vi "feed_forward.vi"(0 "Desired tension velocities [N/s]":dbl[](array[numeric]), 4 "frictionCompensationTensions":dbl[](array[numeric])=[30.0, 30.0, 30.0, 30.0, 30.0, 30.0, 30.0, 30.0, 30.0, 30.0, 30.0, 30.0, 30.0, 30.0], 5 "Use pull-only friction compensation in feedforward":bool, 6 "Motor velocities (rpm)":dbl[](array[numeric]), 7 "DesiredTensionsInAscendingMotorOrder":dbl[](array[numeric]), 8 "Use linear tension/current modle in feedforward":bool, 9 "Num Total Active Motors":i32, 10 "lastCommandedMotorCurrent":dbl[](array[numeric]), 11 "Constants LL":T1) -> (3 "feedforwardPredictedMotorCurrents":dbl[](array[numeric]))   [LabVIEW 2024]
uses:
  typeDef/constants_LL.ctl
panel:
  in  "motor velocity friction comp exponent denominator (rpm)":dbl=50.0
  # "FRICTION COMPENSATION \nVALUES BELOW. \nNOTE: Friction Comp tensions \nare passed in from outside."
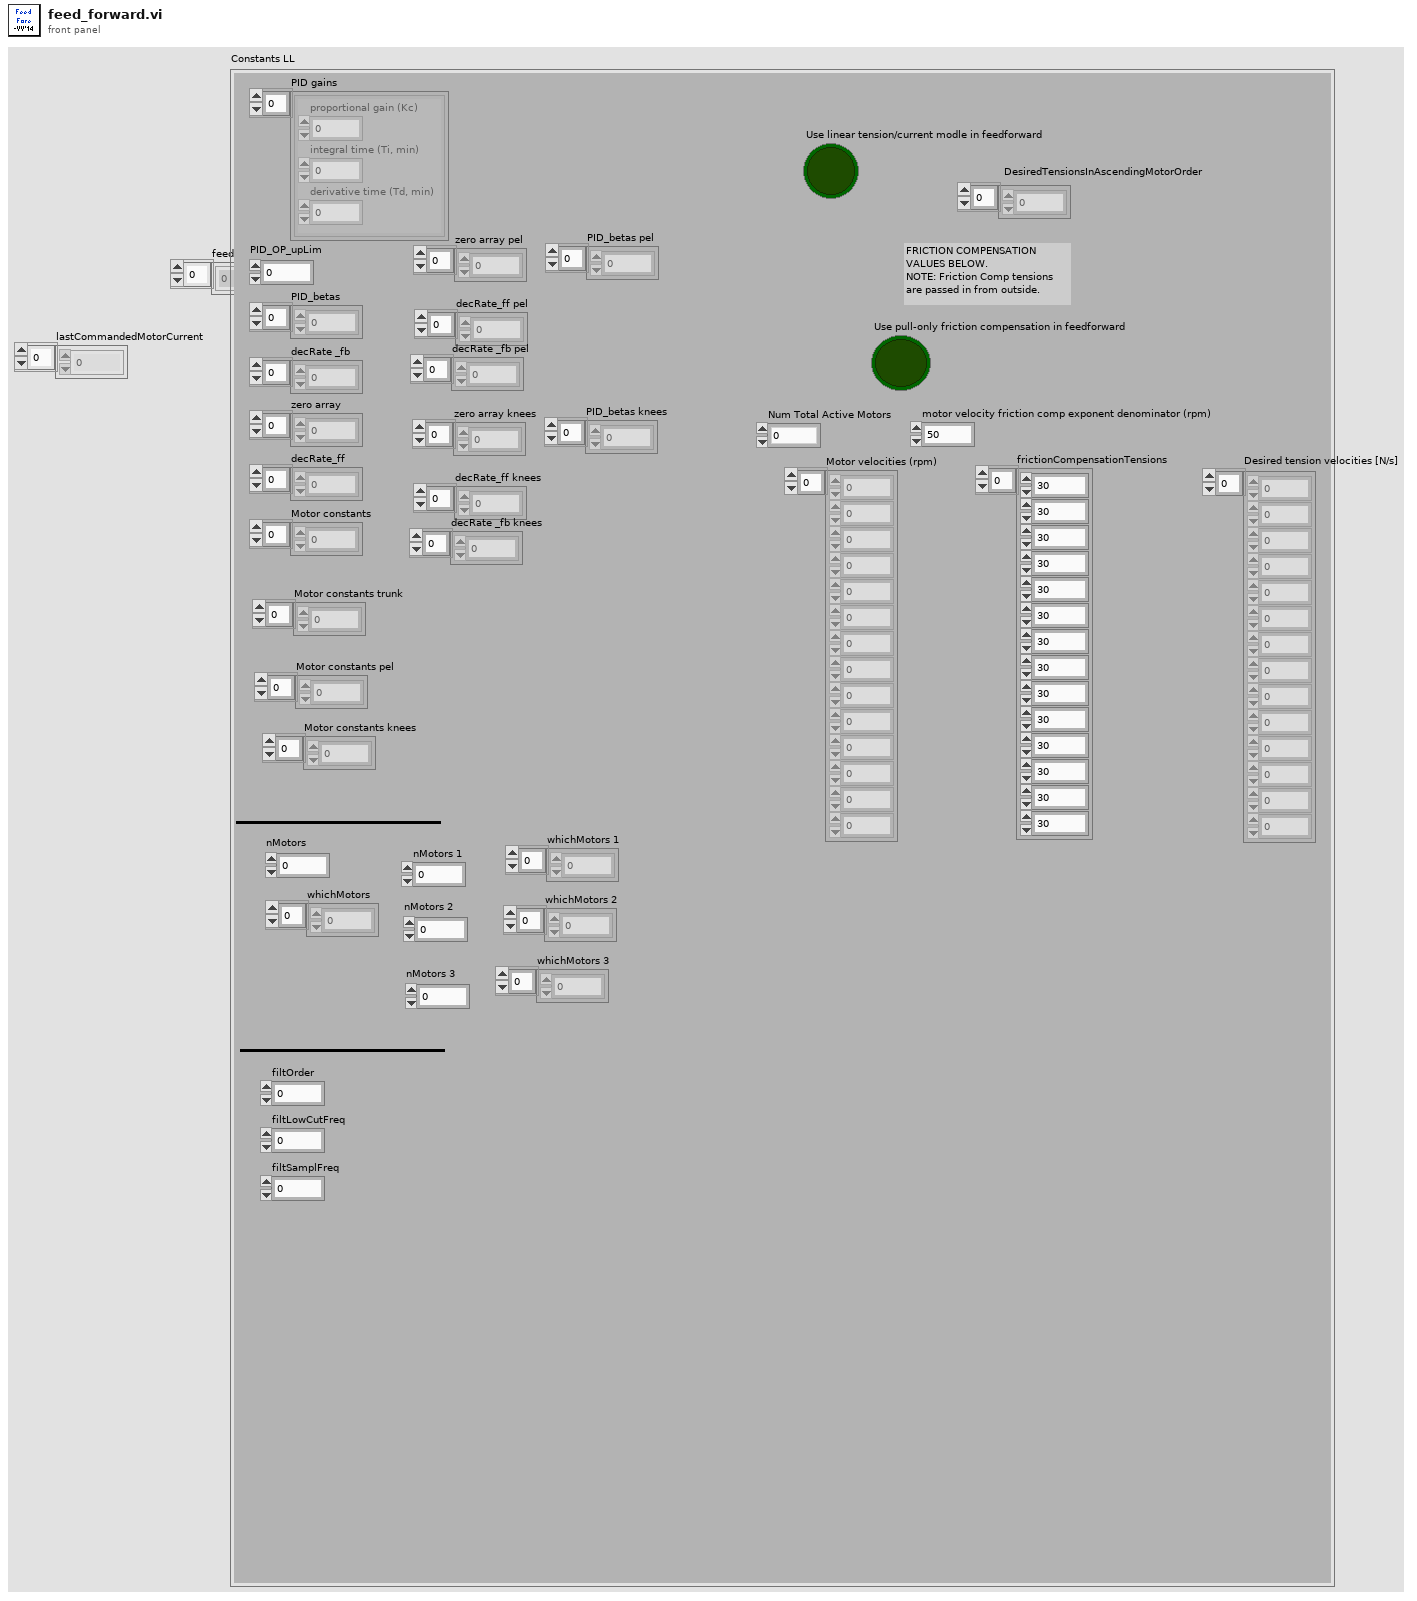
[diagram p1: front panel]
types:
  T1 = typedef "constants_LL.ctl" = cluster{"zero array":dbl[], "decRate_ff":dbl[], "Motor constants":dbl[], "PID gains":cluster{"proportional gain (Kc)":dbl, "integral time (Ti, min)":dbl, "derivative time (Td, min)":dbl}[], "decRate _fb":dbl[], "PID_OP_upLim":dbl, "nMotors":i32, "PID_betas":dbl[], "filtOrder":i32, "filtLowCutFreq":dbl, "filtSamplFreq":dbl, "whichMotors":i32[], "nMotors 1":i32, "nMotors 2":i32, "Motor constants pel":dbl[], "Motor constants trunk":dbl[], "whichMotors 1":i32[], "whichMotors 2":i32[], "zero array pel":dbl[], "decRate_ff pel":dbl[], "decRate _fb pel":dbl[], "PID_betas pel":dbl[], "whichMotors 3":i32[], "nMotors 3":i32, "Motor constants knees":dbl[], "zero array knees":dbl[], "decRate_ff knees":dbl[], "decRate _fb knees":dbl[], "PID_betas knees":dbl[]}
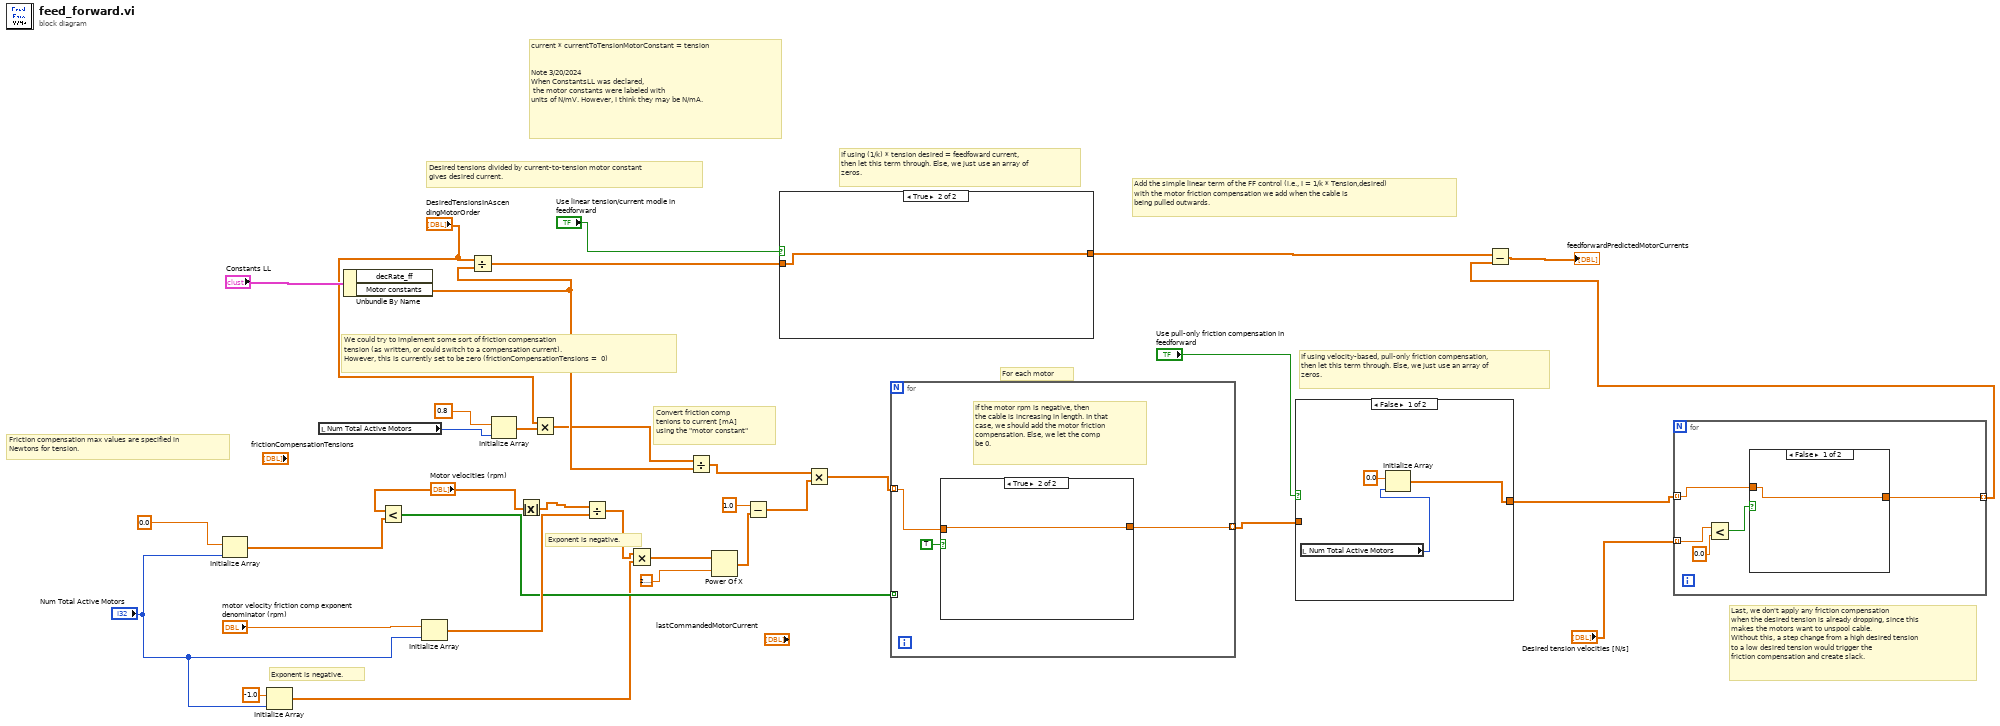
[diagram p0: block diagram]
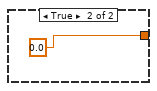
[diagram p2: hidden frame]
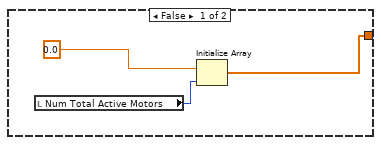
[diagram p4: hidden frame]
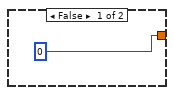
[diagram p5: hidden frame]
diagram:
  # "Last, we don't apply any friction compensation \nwhen the desired tension is already dropping, since this \nmakes the motors want to unspool cable. \nWithout this, a step change from a high desired tension \nto a low desired tension would trigger the \nfriction compensation and create slack."
  # "Friction compensation max values are specified in \nNewtons for tension."
  # "Convert friction comp\ntenions to current [mA] \nusing the \"motor constant\""
  # "If using velocity-based, pull-only friction compensation, \nthen let this term through. Else, we just use an array of \nzeros."
  # "Exponent is negative."
  # "Exponent is negative."
  # "If using (1/k) * tension desired = feedfoward current, \nthen let this term through. Else, we just use an array of \nzeros."
  # "Add the simple linear term of the FF control (i.e., I = 1/k * Tension,desired)\nwith the motor friction compensation we add when the cable is \nbeing pulled outwards."
  # "For each motor"
  # "We could try to implement some sort of friction compensation \ntension (as written, or could switch to a compensation current). \nHowever, this is currently set to be zero (frictionCompensationTensions =  0)"
  # "current * currentToTensionMotorConstant = tension\n\n\nNote 3/20/2024\nWhen ConstantsLL was declared,\n the motor constants were labeled with\nunits of N/mV. However, I think they may be N/mA."
  # "Desired tensions divided by current-to-tension motor constant\ngives desired current."
  n1 = Initialize Array(0.0 ("element"), "Num Total Active Motors") -> (w28:dbl[])
  n2 = Initialize Array(-1.0 ("element"), "Num Total Active Motors") -> (w17:dbl[])
  n3 = local read "Num Total Active Motors"() -> (w10:i32)
  n4 = Unbundle By Name("Constants LL") -> ("Motor constants"=w33:dbl[])  [unwired: 1 out]
  n5 = Less?(x="Motor velocities (rpm)", y=w28) -> (x < y?=w23:bool[])
  n6 = Initialize Array("motor velocity friction comp exponent denominator (rpm)", "Num Total Active Motors") -> (w30:dbl[])
  n7 = Divide(x="DesiredTensionsInAscendingMotorOrder", y=w33) -> (x/y=w21:dbl[])
  n8 = Initialize Array(0.8 ("element"), w10) -> (w8:dbl[])
  n9 = Absolute Value(x="Motor velocities (rpm)") -> (abs(x)=w26:dbl[])
  n10 = Multiply(x="DesiredTensionsInAscendingMotorOrder", y=w8) -> (x*y=w7:dbl[])
  n11 = Divide(x=w26, y=w30) -> (x/y=w20:dbl[])
  n12 = Multiply(x=w20, y=w17) -> (x*y=w16:dbl[])
  n13 = Divide(x=w7, y=w33) -> (x/y=w25:dbl[])
  n14 = Power Of X(1:2.718281828459045, 2:w16) -> (0:w5:dbl[])
  n15 = Subtract(x=1.0, y=w5) -> (x-y=w4:dbl[])
  n16 = case shown="True" "Use linear tension/current modle in feedforward" {
    tunnel: w21 -> [_ w38]
    tunnel: [w35 w38] -> w13
    frame False {
      n17 = local read "Num Total Active Motors"() -> (w36:i32)
      n18 = Initialize Array(0.0 ("element"), w36) -> (w35:dbl[])
    }
    frame True {
    }
  }
  n19 = Multiply(x=w25, y=w4) -> (x*y=w24:dbl[])
  n20 = for {
    tunnel: w24 -> [w41] mode=indexing
    tunnel: w23 -> [_] mode=indexing
    tunnel: [w40] -> w14 mode=indexing
    # "If the motor rpm is negative, then \nthe cable is increasing in length. In that\ncase, we should add the motor friction\ncompensation. Else, we let the comp \nbe 0."
    n21 = case shown="True" TRUE {
      tunnel: w41 -> [_ w43]
      tunnel: [0 w43] -> w40
      frame False {
      }
      frame True {
      }
    }
  }
  n22 = case shown="False" "Use pull-only friction compensation in feedforward" {
    tunnel: w14 -> [_ w47]
    tunnel: [w44 w47] -> w3
    frame False {
      n23 = local read "Num Total Active Motors"() -> (w45:i32)
      n24 = Initialize Array(0.0 ("element"), w45) -> (w44:dbl[])
    }
    frame True {
    }
  }
  n25 = for {
    tunnel: w3 -> [w49] mode=indexing
    tunnel: "Desired tension velocities [N/s]" -> [w52] mode=indexing
    tunnel: [w48] -> w1 mode=indexing
    n26 = Less?(x=w52, y=0.0) -> (x < y?=w50:bool)
    n27 = case shown="False" w50 {
      tunnel: w49 -> [w53 _]
      tunnel: [w53 0.0] -> w48
      frame False {
      }
      frame True {
      }
    }
  }
  n28 = Subtract(x=w13, y=w1) -> (x-y=→"feedforwardPredictedMotorCurrents":dbl[])
